vi "Check Is Menu Button.vi"(10 "Menu Reference":refnum<vi>, 11 "MenuButton in":refnum<class "MenuButton.lvclass">) -> (2 "Is this Menu Button?":bool, 3 "MenuButton out":refnum<class "MenuButton.lvclass">)   [LabVIEW 2017, in "MenuButtons.lvlib" / "MenuButton.lvclass"]
uses:
  MenuButton.lvclass
  MenuButton.lvclass/MenuButton.ctl
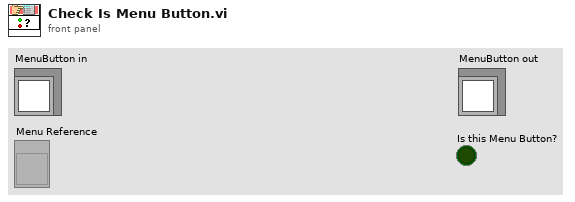
[diagram p1: front panel]
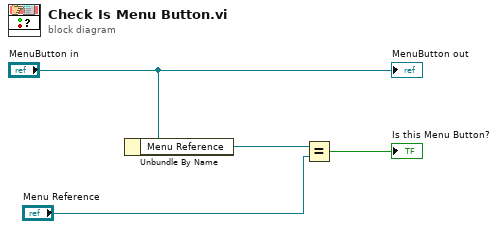
[diagram p0: block diagram]
diagram:
  n1 = Unbundle By Name("MenuButton in") -> ("Menu Reference"=w3:refnum<vi>)
  n2 = Equal?(x=w3, y="Menu Reference") -> (x = y?=→"Is this Menu Button?":bool)
  "MenuButton out" <- "MenuButton in"
